vi "Refresh.vi"(8 "error in (no error)":errorcluster, 10 "Debug Log":T1[](array[typedef]), 11 "Debug Log View In":refnum<class "Debug Log View.lvclass">) -> (0 "error out":errorcluster, 3 "Debug Log View Out":refnum<class "Debug Log View.lvclass">)   [LabVIEW 2020, in "Debug Log View.lvclass"]
uses:
  Debug Log View.lvclass
  Debugger/TypeDefs/Debug Data.ctl
  Debugger/Debugger.lvclass
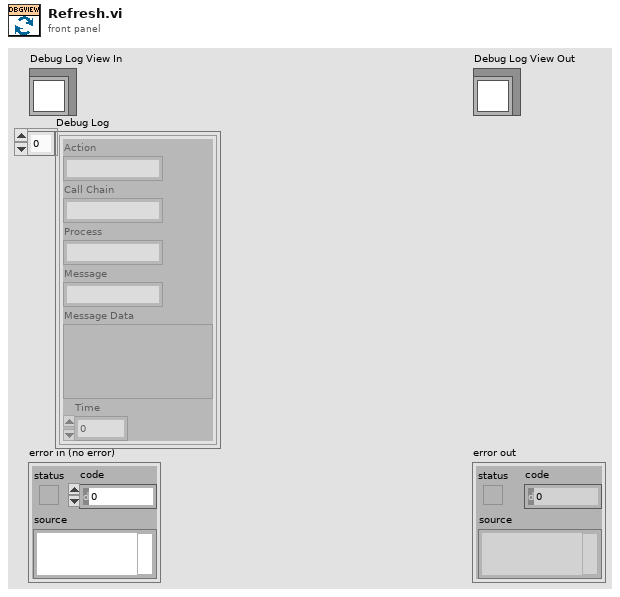
[diagram p1: front panel]
types:
  T1 = typedef "Debugger.lvclass/Debug Data.ctl" = cluster{"Action":string, "Call Chain":string, "Process":string, "Message":string, "Message Data":variant, "Time":u32}
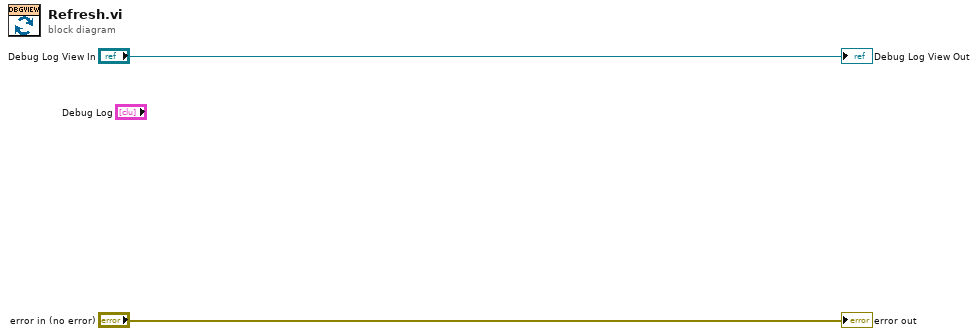
[diagram p0: block diagram]
diagram:
  "error out" <- "error in (no error)"
  "Debug Log View Out" <- "Debug Log View In"
